vi "Get Control Image.vi"(8 "error in (no error)":errorcluster, 11 "Control ref":refnum<vi>) -> (0 "error out":errorcluster, 2 "All base64 Images":string[](array[string]), 3 "base64 encoded <img>":string)   [LabVIEW 2015, in "Front Panel Publisher.lvlib" / "Control.lvclass"]
uses:
  Control.lvclass
  Front Panel Publisher.lvlib
  <vilib>/wsapi/NI_WebServices.lvlib
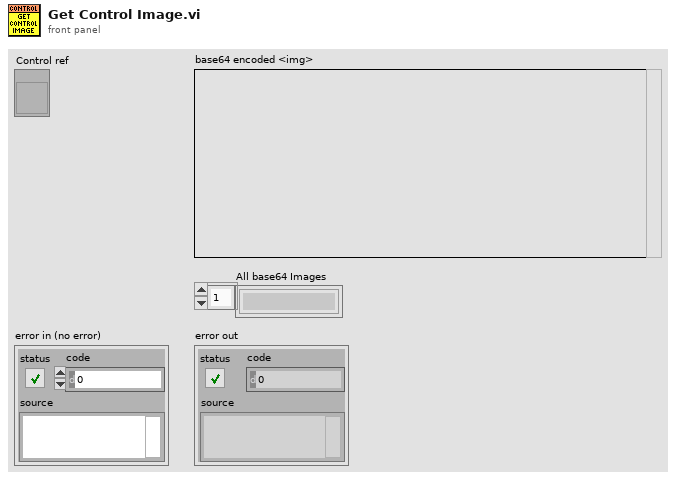
[diagram p1: front panel]
types:
  T1 = typedef "imagedata.ctl" = cluster{"image type":i32, "image depth":i32, "image":u8[], "mask":u8[], "colors":u32[], "Rectangle":cluster{"left":i16, "top":i16, "right":i16, "bottom":i16}}
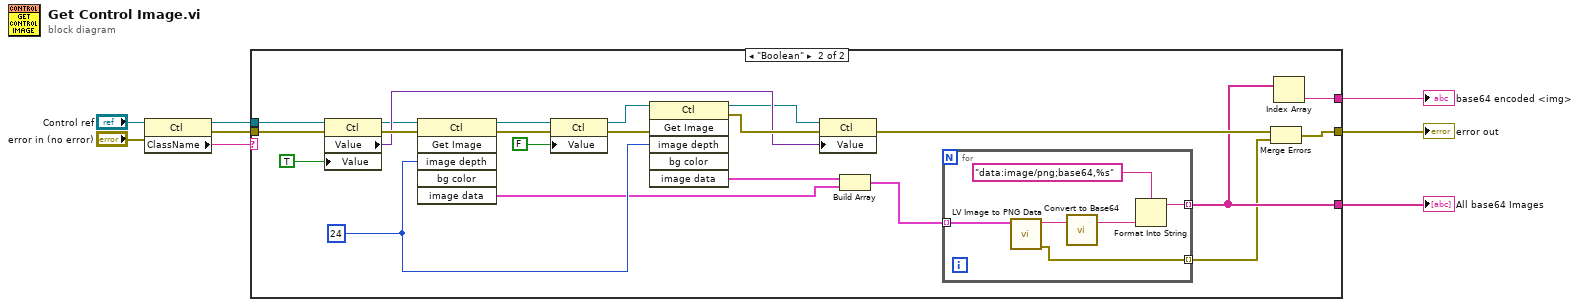
[diagram p0: block diagram]
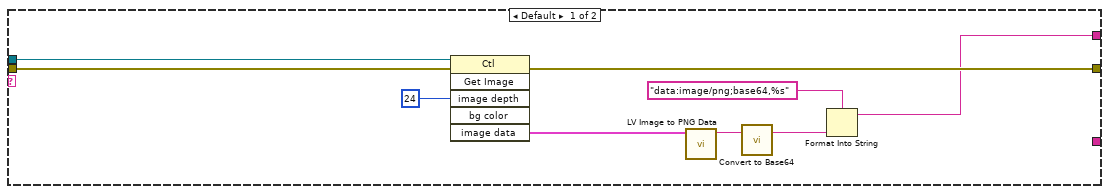
[diagram p2: hidden frame]
diagram:
  n1 = property on="Property Node" class="Ctl"(reference="Control ref", error in="error in (no error)") -> (reference out=w4:refnum<vi>, error out=w7:errorcluster, "ClassName"=w3:string)
  n2 = case shown="\"Boolean\"" w3 {
    tunnel: [_ w21] -> w1
    tunnel: [w16 w19] -> w6
    tunnel: w4 -> [w14 w25]
    tunnel: w7 -> [w17 w34]
    tunnel: [w9 w20] -> w2
    frame Default {
      n3 = invoke on="Invoke Node" class="Ctl" method="Get Image"(reference=w14, error in=w17, "image depth"=24 ("Image Depth")) -> (error out=w16:errorcluster, "image data"=w11:T1)  [unwired: 3 in, 4 out]
      n4 = call <vilib>:"LV Image to PNG Data.vi"("image data"=w11) -> ("png data"=w13:string)  [unwired: 9 in, 1 out]
      n5 = call "Convert to Base64.vi"("String"=w13) -> ("Base64 String"=w12:string)  [unwired: 2 in]
      n6 = Format Into String(format string="data:image/png;base64,%s" ("string"), w12) -> (resulting string=w9:string)  [unwired: 2 in, 1 out]
    }
    frame "Boolean" {
      w26 = 24 ("Image Depth")
      n7 = property on="Property Node" class="Ctl"(reference=w25, error in=w34, "Value"=TRUE) -> (reference out=w30:refnum<vi>, error out=w36:errorcluster, "Value"=w33:variant)
      n8 = invoke on="Invoke Node" class="Ctl" method="Get Image"(reference=w30, error in=w36, "image depth"=w26) -> (reference out=w29:refnum<vi>, error out=w37:errorcluster, "image data"=w23:T1)  [unwired: 3 in, 3 out]
      n9 = property on="Property Node" class="Ctl"(reference=w29, error in=w37, "Value"=FALSE) -> (reference out=w32:refnum<vi>, error out=w39:errorcluster)
      n10 = invoke on="Invoke Node" class="Ctl" method="Get Image"(reference=w32, error in=w39, "image depth"=w26) -> (reference out=w31:refnum<vi>, error out=w38:errorcluster, "image data"=w24:T1)  [unwired: 3 in, 3 out]
      n11 = property on="Property Node" class="Ctl"(reference=w31, error in=w38, "Value"=w33) -> (error out=w35:errorcluster)  [unwired: 1 out]
      n12 = Build Array(w24, w23) -> (w22:T1[])
      n13 = for {
        tunnel: w22 -> [w42] mode=indexing
        tunnel: [w41] -> w21 mode=indexing
        tunnel: [w40] -> w18 mode=indexing
        n14 = call <vilib>:"LV Image to PNG Data.vi"("image data"=w42) -> ("error out"=w40:errorcluster, "png data"=w43:string)  [unwired: 9 in]
        n15 = call "Convert to Base64.vi"("String"=w43) -> ("Base64 String"=w45:string)  [unwired: 2 in]
        n16 = Format Into String(format string="data:image/png;base64,%s" ("string"), w45) -> (resulting string=w41:string)  [unwired: 2 in, 1 out]
      }
      n17 = Merge Errors(w35, w18) -> (w19:errorcluster)
      n18 = Index Array(array=w21) -> (element=w20:string)  [unwired: 1 in]
    }
  }
  "error out" <- w6
  "base64 encoded <img>" <- w2
  "All base64 Images" <- w1
